vi "test ZMQ regex.vi"() -> ()   [LabVIEW 2018]
uses:
  <vilib>/regexp/Match Regular Expression.xnode
panel:
  in  "regular expression":string="{\"msg_type\":\"data\",\"msg_property\":\"Vset\", \"PMT1\" : \"PMTValue1\", \"PMT2\" :\"PMVal2\" }"
  out "error out":errorcluster
  out "remainder":string
  out "Vals":string[](array[string])
  out "property":string[](array[string])
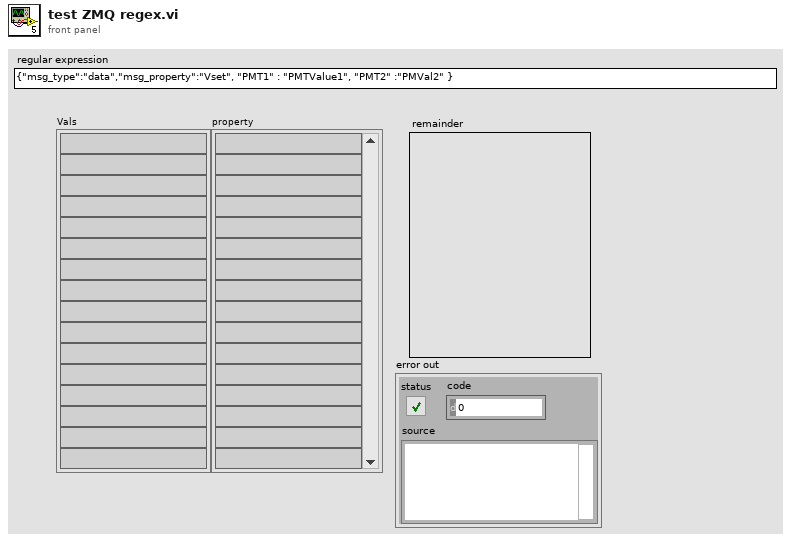
[diagram p1: front panel]
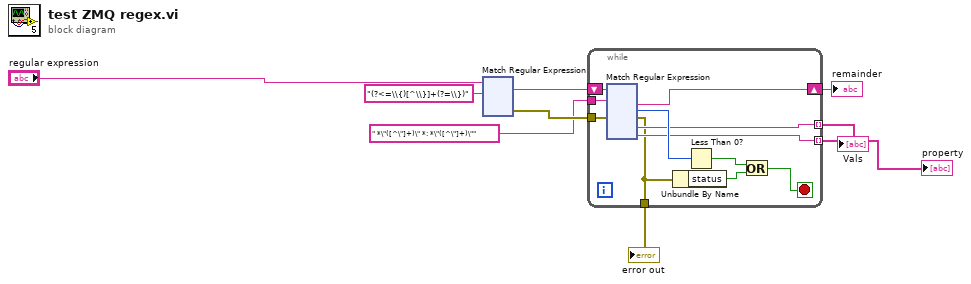
[diagram p0: block diagram]
diagram:
  n1 = xnode "Match Regular Expression"("input string"="regular expression", "regular expression"="(?<=\\{)[^\\}]+(?=\\})") -> ("whole match"=w6:string, "error out"=w7:errorcluster)  [unwired: 4 in, 3 out]
  n2 = while {
    tunnel: w7 -> [w17]
    tunnel: " *\"([^\"]+)\" *: *\"([^\"]+)\"" ("regular expression") -> [w15]
    tunnel: [w13] -> w4 mode=indexing
    tunnel: [w12] -> w3 mode=indexing
    shift-right: [w11] -> w2
    shift-left: w6 -> [w16]
    tunnel: [w10] -> w1
    stop <- w14 stop-if-true
    n3 = xnode "Match Regular Expression"("input string"=w16, "regular expression"=w15, "error in"=w17) -> ("after match"=w11:string, "offset past match"=w20:i32, "error out"=w10:errorcluster, "submatch 1"=w12:string, "submatch 2"=w13:string)  [unwired: 3 in, 2 out]
    n4 = Unbundle By Name(w10) -> ("status"=w18:bool)
    n5 = Less Than 0?(x=w20) -> (x < 0?=w19:bool)
    n6 = Or(x=w19, y=w18) -> (x .or. y?=w14:bool)
  }
  "property" <- w4
  "Vals" <- w3
  "remainder" <- w2
  "error out" <- w1
